vi "Change Desired Temperature.vi"(8 "error in (no error)":errorcluster, 10 "Desired Temperture":dbl, 11 "Cooler UI with Events in":refnum<class "Cooler UI with Events.lvclass">) -> (0 "error out":errorcluster, 3 "Cooler UI with Events out":refnum<class "Cooler UI with Events.lvclass">)   [LabVIEW 2012, in "Cooler UI.lvlib" / "Cooler UI with Events.lvclass"]
uses:
  Cooler UI with Events.lvclass
  Cooler UI with Events.lvclass/Cooler UI with Events.ctl
  Level Controller/Level Controller Messages/Write Deadband Msg/Write Deadband Msg.lvclass/Write Deadband Msg.ctl
  <vilib>/ActorFramework/Message Enqueuer/Message Enqueuer.lvclass/Message Enqueuer.ctl
  <vilib>/ActorFramework/Message Enqueuer/Enqueue.vi
  <vilib>/ActorFramework/Message Priority Queue/Priority Enqueue.vi
  Level Controller/Level Controller Messages/Write Deadband Msg/Write Deadband Msg.lvclass
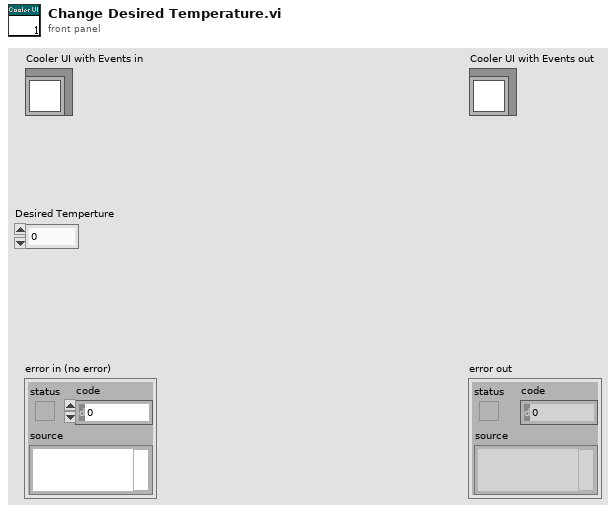
[diagram p1: front panel]
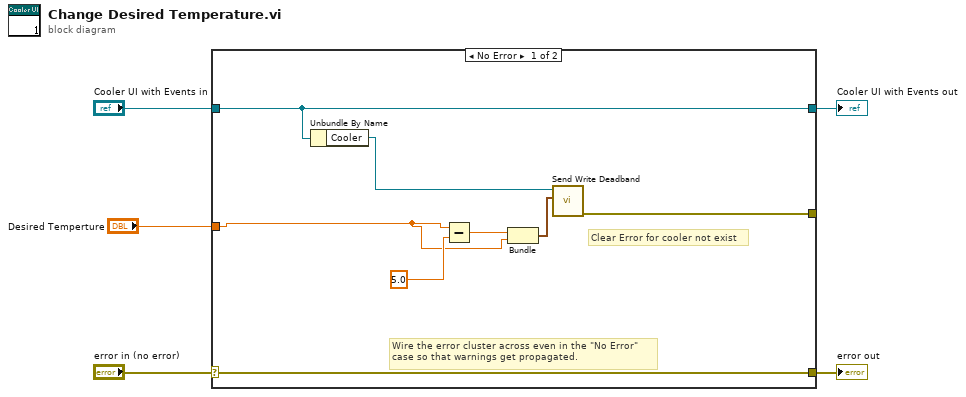
[diagram p0: block diagram]
diagram:
  n1 = case shown="No Error" "error in (no error)" {
    selector: "error in (no error)" -> [w13 w15]
    tunnel: [w13 w15] -> w4
    tunnel: [w12 w14] -> w2
    tunnel: "Cooler UI with Events in" -> [w12 w14]
    tunnel: "Desired Temperture" -> [w7 _]
    tunnel: [w6 _] -> _
    frame No Error {
      # "Clear Error for cooler not exist"
      # "Wire the error cluster across even in the \"No Error\"\ncase so that warnings get propagated."
      n2 = Unbundle By Name(w12) -> ("Cooler"=w11:refnum<class "Message Enqueuer.lvclass">)
      n3 = Subtract(x=w7, y=5.0) -> (x-y=w8:dbl)
      n4 = Bundle(w8, "Desired Temperture"=w7) -> (w10:cluster{dbl, "Desired Temperture":dbl})  [unwired: 1 in]
      n5 = call "Send Write Deadband.vi"("Deadband"=w10, "Message Enqueuer"=w11) -> ("error out"=w6:errorcluster)  [unwired: 8 in, 1 out]
    }
    frame Error {
    }
  }
  "error out" <- w4
  "Cooler UI with Events out" <- w2
